vi "sub_GSlam_fill-Hnb.vi"(9 "edge":T2, 10 "b":T1, 11 "H":T1) -> (2 "b out":T1 caption="b", 3 "H out":T1 caption="H")   [LabVIEW 2019]
uses:
  <vilib>/Analysis/Matrix/Datatypes/RealMatrix.ctl
  Ctrl/cmd_common.ctl
  <vilib>/Analysis/Matrix/Numeric/Multiply/Multiply - RM,RM.vi
  <vilib>/Analysis/Matrix/Numeric/Add/Add - RM,RM.vi
  <vilib>/Analysis/Matrix/NI_Matrix.lvlib
panel:
  out "열의 개수 2":i32
  out "행의 개수 2":i32
  out "열의 개수":i32
  out "행의 개수":i32
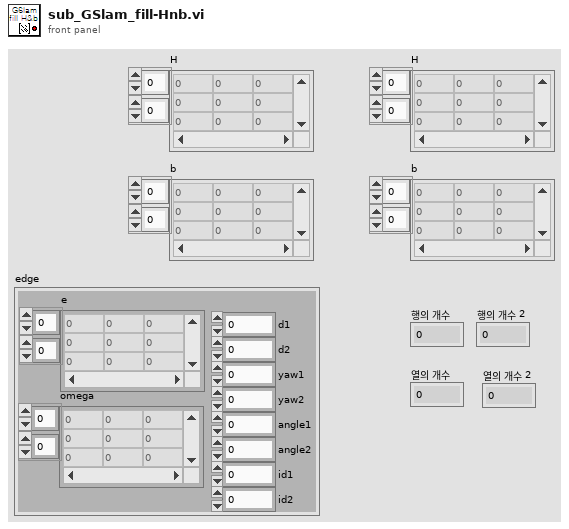
[diagram p1: front panel]
types:
  T1 = typedef "NI_Matrix.lvlib/RealMatrix.ctl" = dbl[][]
  T2 = cluster{"e":T1, "omega":T1, "d1":dbl, "d2":dbl, "yaw1":dbl, "yaw2":dbl, "angle1":dbl, "angle2":dbl, "id1":i32, "id2":i32}
  T3 = typedef "cmd_common.ctl" = enum16{"read", "write"}
  T4 = cluster{"Q Sim":T1, "R Sim":T1, "DT":dbl, "SIM_TIME":dbl, "MAX_RANGE":dbl, "STATE_SIZE":i32, "C_SIGMA 1":dbl, "C_SIGMA 2":dbl, "C_SIGMA 3":dbl, "MAX_ITR":u32}
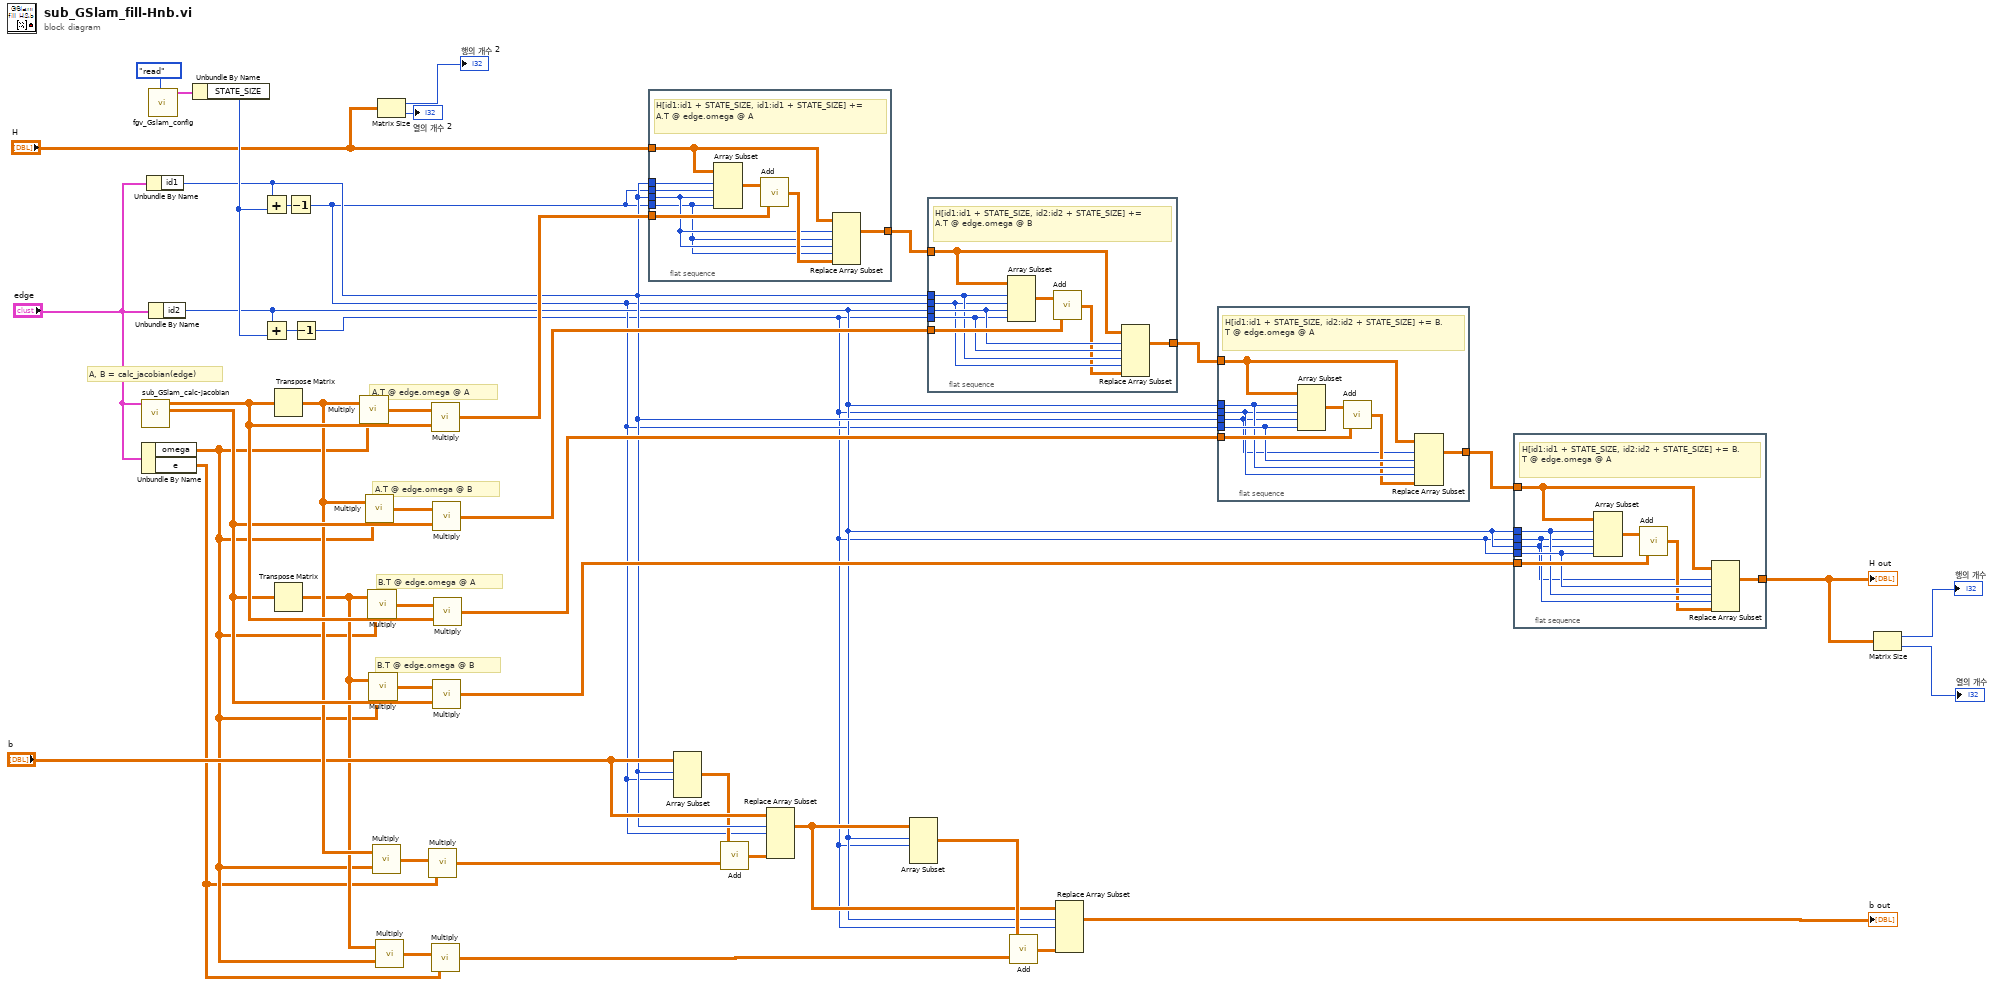
[diagram p0: block diagram]
diagram:
  # "B.T @ edge.omega @ B"
  # "B.T @ edge.omega @ A"
  # "A.T @ edge.omega @ B"
  # "A, B = calc_jacobian(edge)"
  # "A.T @ edge.omega @ A"
  n1 = call "sub_GSlam_calc-jacobian.vi"("edge"="edge") -> ("B"=w33:T1, "A"=w34:T1)  [unwired: 9 in]
  n2 = Unbundle By Name("edge") -> ("omega"=w15:T1, "e"=w14:T1)
  n3 = Unbundle By Name("edge") -> ("id1"=w24:i32)
  n4 = call "fgv_Gslam_config.vi"("cmd"=cmd_common."read") -> ("G cofnig out"=w43:T4)  [unwired: 10 in]
  n5 = Unbundle By Name("edge") -> ("id2"=w11:i32)
  n6 = Unbundle By Name(w43) -> ("STATE_SIZE"=w42:i32)
  n7 = Add(x=w24, y=w42) -> (x+y=w23:i32)
  n8 = Add(x=w11, y=w42) -> (x+y=w10:i32)
  n9 = Transpose Matrix(1:w34) -> (0:w27:T1)
  n10 = Transpose Matrix(1:w33) -> (0:w16:T1)
  n11 = Decrement(x=w23) -> (x-1=w8:i32)
  n12 = Decrement(x=w10) -> (x-1=w7:i32)
  n13 = call-poly <vilib>:"Multiply.vi"("Real Matrix B"=w15, "Real Matrix A"=w27) -> ("A * B"=w41:T1)
  n14 = call-poly <vilib>:"Multiply.vi"("Real Matrix B"=w15, "Real Matrix A"=w27) -> ("A * B"=w38:T1)
  n15 = call-poly <vilib>:"Multiply.vi"("Real Matrix B"=w15, "Real Matrix A"=w16) -> ("A * B"=w36:T1)
  n16 = call-poly <vilib>:"Multiply.vi"("Real Matrix B"=w15, "Real Matrix A"=w16) -> ("A * B"=w35:T1)
  n17 = call-poly <vilib>:"Multiply.vi"("Real Matrix B"=w15, "Real Matrix A"=w27) -> ("A * B"=w26:T1)
  n18 = call-poly <vilib>:"Multiply.vi"("Real Matrix B"=w15, "Real Matrix A"=w16) -> ("A * B"=w17:T1)
  n19 = Matrix Size(0:"H") -> (1:→"행의 개수 2":i32, 2:→"열의 개수 2":i32)
  n20 = call-poly <vilib>:"Multiply.vi"("Real Matrix B"=w14, "Real Matrix A"=w26) -> ("A * B"=w21:T1)
  n21 = call-poly <vilib>:"Multiply.vi"("Real Matrix B"=w34, "Real Matrix A"=w41) -> ("A * B"=w39:T1)
  n22 = call-poly <vilib>:"Multiply.vi"("Real Matrix B"=w14, "Real Matrix A"=w17) -> ("A * B"=w13:T1)
  n23 = call-poly <vilib>:"Multiply.vi"("Real Matrix B"=w33, "Real Matrix A"=w38) -> ("A * B"=w37:T1)
  n24 = call-poly <vilib>:"Multiply.vi"("Real Matrix B"=w33, "Real Matrix A"=w35) -> ("A * B"=w28:T1)
  n25 = call-poly <vilib>:"Multiply.vi"("Real Matrix B"=w34, "Real Matrix A"=w36) -> ("A * B"=w30:T1)
  n26 = flat-sequence {
    tunnel: w39 -> [w52]
    tunnel: "H" -> [w51]
    tunnel: w24 -> [w48]
    tunnel: w8 -> [w45]
    tunnel: [w49] -> w32
    tunnel: w24 -> [w47]
    tunnel: w8 -> [w46]
    frame #0 {
      # "H[id1:id1 + STATE_SIZE, id1:id1 + STATE_SIZE] += A.T @ edge.omega @ A"
      n27 = Array Subset(array=w51, index (row)=w47, length (row)=w46, index (col)=w48, length (col)=w45) -> (w53:T1)
      n28 = call-poly <vilib>:"Add.vi"("Real Matrix B"=w52, "Real Matrix A"=w53) -> ("A + B"=w50:T1)
      n29 = Replace Array Subset(array=w51, new element=w50, index (dim 0)=w48, index (dim 1)=w45, index (dim 2)=w48, index (dim 3)=w45) -> (w49:T1)
    }
  }
  n30 = Array Subset(array="b", index (row)=w24, length (row)=w8) -> (w22:T1)  [unwired: 2 in]
  n31 = call-poly <vilib>:"Add.vi"("Real Matrix B"=w21, "Real Matrix A"=w22) -> ("A + B"=w20:T1)
  n32 = Replace Array Subset(array="b", new element=w20, index (dim 0)=w24, index (dim 1)=w8) -> (w12:T1)  [unwired: 2 in]
  n33 = Array Subset(array=w12, index (row)=w11, length (row)=w7) -> (w18:T1)  [unwired: 2 in]
  n34 = flat-sequence {
    tunnel: w37 -> [w61]
    tunnel: w11 -> [w60]
    tunnel: w7 -> [w59]
    tunnel: w24 -> [w58]
    tunnel: w8 -> [w57]
    tunnel: [w56] -> w31
    tunnel: w32 -> [w54]
    frame #0 {
      # "H[id1:id1 + STATE_SIZE, id2:id2 + STATE_SIZE] += A.T @ edge.omega @ B"
      n35 = Array Subset(array=w54, index (row)=w58, length (row)=w57, index (col)=w60, length (col)=w59) -> (w62:T1)
      n36 = call-poly <vilib>:"Add.vi"("Real Matrix B"=w61, "Real Matrix A"=w62) -> ("A + B"=w55:T1)
      n37 = Replace Array Subset(array=w54, new element=w55, index (dim 0)=w60, index (dim 1)=w59, index (dim 2)=w58, index (dim 3)=w57) -> (w56:T1)
    }
  }
  n38 = call-poly <vilib>:"Add.vi"("Real Matrix B"=w13, "Real Matrix A"=w18) -> ("A + B"=w19:T1)
  n39 = Replace Array Subset(array=w12, new element=w19, index (dim 0)=w11, index (dim 1)=w7) -> (→"b out":T1)  [unwired: 2 in]
  n40 = flat-sequence {
    tunnel: w30 -> [w70]
    tunnel: [w63] -> _
    tunnel: w8 -> [w69]
    tunnel: w11 -> [w68]
    tunnel: w7 -> [w67]
    tunnel: [w66] -> w29
    tunnel: w31 -> [w64]
    tunnel: w24 -> [w63]
    frame #0 {
      # "H[id1:id1 + STATE_SIZE, id2:id2 + STATE_SIZE] += B.T @ edge.omega @ A"
      n41 = Array Subset(array=w64, index (row)=w68, length (row)=w67, index (col)=w63, length (col)=w69) -> (w71:T1)
      n42 = call-poly <vilib>:"Add.vi"("Real Matrix B"=w70, "Real Matrix A"=w71) -> ("A + B"=w65:T1)
      n43 = Replace Array Subset(array=w64, new element=w65, index (dim 0)=w63, index (dim 1)=w69, index (dim 2)=w68, index (dim 3)=w67) -> (w66:T1)
    }
  }
  n44 = flat-sequence {
    tunnel: w28 -> [w79]
    tunnel: w11 -> [w72]
    tunnel: w7 -> [w78]
    tunnel: w11 -> [w77]
    tunnel: w7 -> [w76]
    tunnel: [w75] -> w6
    tunnel: w29 -> [w73]
    tunnel: [w72] -> _
    frame #0 {
      # "H[id1:id1 + STATE_SIZE, id2:id2 + STATE_SIZE] += B.T @ edge.omega @ A"
      n45 = Array Subset(array=w73, index (row)=w77, length (row)=w76, index (col)=w72, length (col)=w78) -> (w80:T1)
      n46 = call-poly <vilib>:"Add.vi"("Real Matrix B"=w79, "Real Matrix A"=w80) -> ("A + B"=w74:T1)
      n47 = Replace Array Subset(array=w73, new element=w74, index (dim 0)=w72, index (dim 1)=w78, index (dim 2)=w77, index (dim 3)=w76) -> (w75:T1)
    }
  }
  n48 = Matrix Size(0:w6) -> (1:→"행의 개수":i32, 2:→"열의 개수":i32)
  "H out" <- w6
